vi "Integral Stabilization.vi"() -> ()   [LabVIEW 2010]
uses:
  Global Variables/Global Stop.vi
panel:
  in  "Activate Output":bool
  in  "Integration Time Interval":dbl=300.0
  in  "Reset Integral":bool
  out "Thick Etalon Pos Setp on Activation":i32
  out "Wavenumber on Activation":dbl format="%.4f"
  in  "Correction Output":bool
  out "correction steps":dbl
  in  "Difference Threshold":dbl=0.05
  in  "Integral Correction Factor":dbl=0.005
  out "New Wavemeter Value":bool
  out "Out of Range":bool
  in  "Stop":bool
  out "PStab loop counter":i32
  in  "Thick Etalon Position Setpoint":i32
  in  "Invert Output":bool=TRUE
  in  "Wavenumber Setpoint":dbl format="%.4f"
  out "WS7 Ch1 Wavenumber":dbl format="%.4f"
  # "Invert Output\nif moving beyond\nFlash Position"
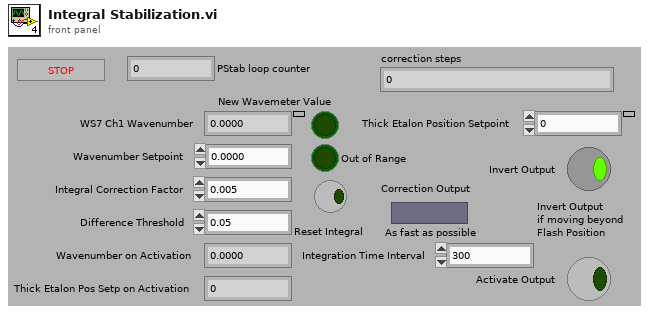
[diagram p1: front panel]
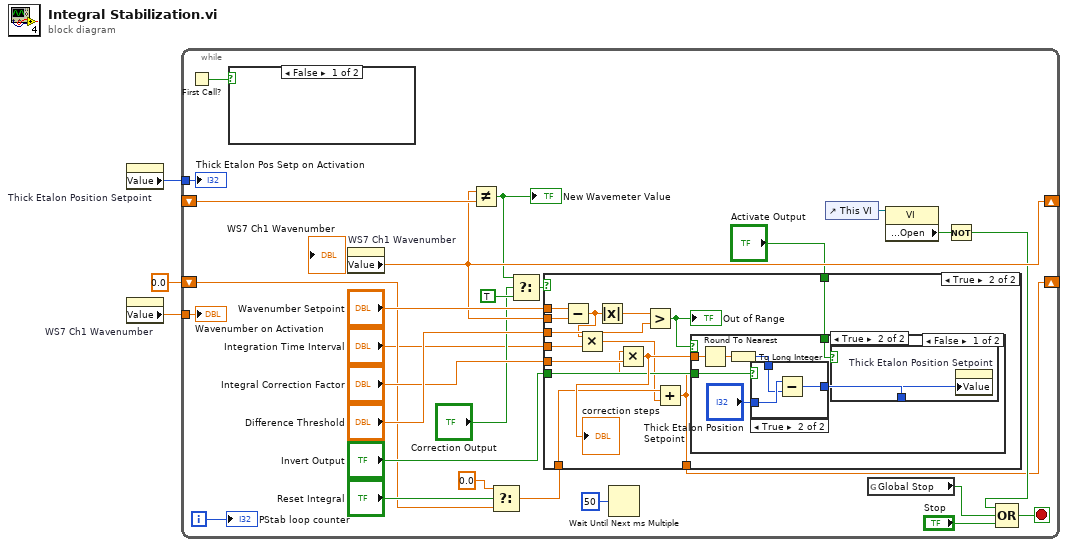
[diagram p0: block diagram]
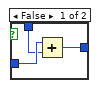
[diagram p4: hidden frame]
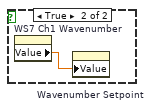
[diagram p6: hidden frame]
diagram:
  n1 = property on="Thick Etalon Position Setpoint" class="DigNum (strict)"() -> ("Value"=w2:i32)  [unwired: 2 in, 2 out]
  n2 = property on="WS7 Ch1 Wavenumber" class="DigNum (strict)"() -> ("Value"=w3:dbl)  [unwired: 2 in, 2 out]
  n3 = while {
    shift-right: [w28] -> _
    shift-left: _ -> [w30]
    tunnel: w3 -> [w12]
    tunnel: w2 -> [w11]
    shift-right: [w5] -> _
    shift-left: 0.0 -> [w8]
    i -> [w26]
    stop <- w16 stop-if-true
    n4 = First Call?() -> (First Call?: T/F=w31:bool)
    n5 = case shown="False" w31 {
      frame False {
      }
      frame True {
        n6 = property on="WS7 Ch1 Wavenumber" class="DigNum (strict)"() -> ("Value"=w61:dbl)  [unwired: 2 in, 2 out]
        n7 = property on="Wavenumber Setpoint" class="DigNum (strict)"("Value"=w61) -> ()  [unwired: 2 in, 2 out]
      }
    }
    n8 = property on="WS7 Ch1 Wavenumber" class="DigNum (strict)"() -> ("Value"=w28:dbl)  [unwired: 2 in, 2 out]
    n9 = Not Equal?(x=w28, y=w30) -> (x != y?=w21:bool)
    "New Wavemeter Value" <- w21
    n10 = Select(t=0.0, s="Reset Integral", f=w8) -> (s? t:f=w6:dbl)
    n11 = Select(t=w21, s="Correction Output", f=TRUE) -> (s? t:f=w22:bool)
    n12 = case shown="True" w22 {
      tunnel: "Wavenumber Setpoint" -> [_ w46]
      tunnel: w28 -> [_ w45]
      tunnel: "Difference Threshold" -> [_ w42]
      tunnel: "Integral Correction Factor" -> [_ w41]
      tunnel: "Invert Output" -> [_ w39]
      tunnel: "Integration Time Interval" -> [_ w37]
      tunnel: w6 -> [w32 w36]
      tunnel: [w32 w34] -> w5
      tunnel: "Activate Output" -> [_ w33]
      frame False {
      }
      frame True {
        n13 = Subtract(x=w46, y=w45) -> (x-y=w38:dbl)
        n14 = Multiply(x=w38, y=w37) -> (x*y=w35:dbl)
        n15 = Absolute Value(x=w38) -> (abs(x)=w44:dbl)
        n16 = Greater?(x=w44, y=w42) -> (0:w43:bool)
        "Out of Range" <- w43
        n17 = Add(x=w36, y=w35) -> (x+y=w34:dbl)
        n18 = Multiply(x=w34, y=w41) -> (x*y=w40:dbl)
        "correction steps" <- w40
        n19 = case shown="False" w43 {
          tunnel: w40 -> [w52 _]
          tunnel: w39 -> [w50 _]
          tunnel: w33 -> [w47 _]
          frame False {
            n20 = Round To Nearest(number=w52) -> (nearest integer value=w49:dbl)
            n21 = To Long Integer(number=w49) -> (32bit integer=w48:i32)
            n22 = case shown="True" w50 {
              tunnel: "Thick Etalon Position Setpoint" -> [w57 w60]
              tunnel: w48 -> [w56 w59]
              tunnel: [w55 w58] -> w51
              frame False {
                n23 = Add(x=w57, y=w56) -> (x+y=w55:i32)
              }
              frame True {
                n24 = Subtract(x=w60, y=w59) -> (x-y=w58:i32)
              }
            }
            n25 = case shown="True" w47 {
              tunnel: w51 -> [_ w54]
              frame False {
              }
              frame True {
                n26 = property on="Thick Etalon Position Setpoint" class="DigNum (strict)"("Value"=w54) -> ()  [unwired: 2 in, 2 out]
              }
            }
          }
          frame True {
          }
        }
      }
    }
    n27 = Wait Until Next ms Multiple(millisecond multiple=u32 50) -> ()  [unwired: 1 out]
    n28 = control-ref of="This VI"() -> (w17:refnum<vi>)
    n29 = global read "Global Stop.vi" "Global Stop"() -> (w14:bool)
    n30 = property class="VI"(reference=w17) -> ("Front Panel.Open"=w18:bool)  [unwired: 1 in, 2 out]
    n31 = Not(x=w18) -> (.not. x?=w15:bool)
    n32 = Compound Arithmetic op=OR(w15, w14, "Stop") -> (w16:bool)
    "PStab loop counter" <- w26
    "Wavenumber on Activation" <- w12
    "Thick Etalon Pos Setp on Activation" <- w11
  }
